vi "sv_Filter Even-Angle Signal for Specific Harmonic.vi"(0 "even-angle signals":cluster{"r0":dbl, "dr":dbl, "Y":dbl[]}[](array[cluster]), 2 "reset?":bool, 7 "even-angle position info":T1, 9 "specific harmonic":dbl=1.0 format="%0.2f", 11 "error in (no error)":errorcluster, 13 "zero delay? (F)":bool) -> (4 "even-angle signals out":cluster{"r0":dbl, "dr":dbl, "Y":dbl[]}[](array[cluster]), 8 "even-angle position info out":T1, 10 "phase delay [1/cycle]":dbl, 15 "error out":errorcluster)   [LabVIEW 2017, in "SoundVib_ContSweptSine.lvlib"]
uses:
  <vilib>/addons/Sound and Vibration/svt_Continuous Swept Sine/SoundVib_ContSweptSine.lvlib
  <vilib>/addons/Sound and Vibration/Order Analysis/Misc/OAT Position Info.ctl
  <vilib>/Analysis/3filter.llb/FIR Filter with I.C. (DBL).vi
  <vilib>/Analysis/NI_AALBase.lvlib
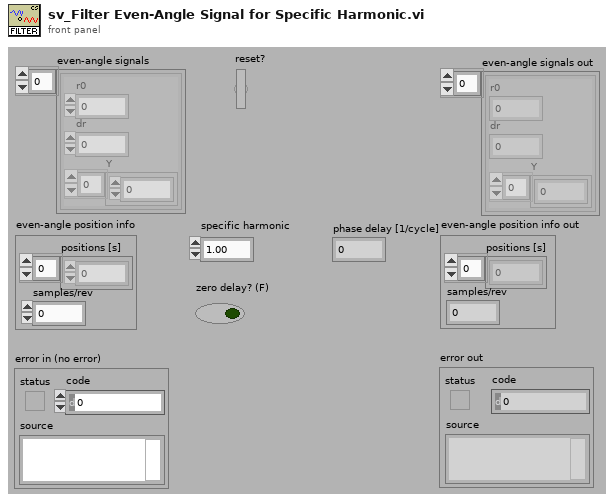
[diagram p1: front panel]
types:
  T1 = typedef "OAT Position Info.ctl" = cluster{"positions [s]":dbl[], "samples/rev":dbl}
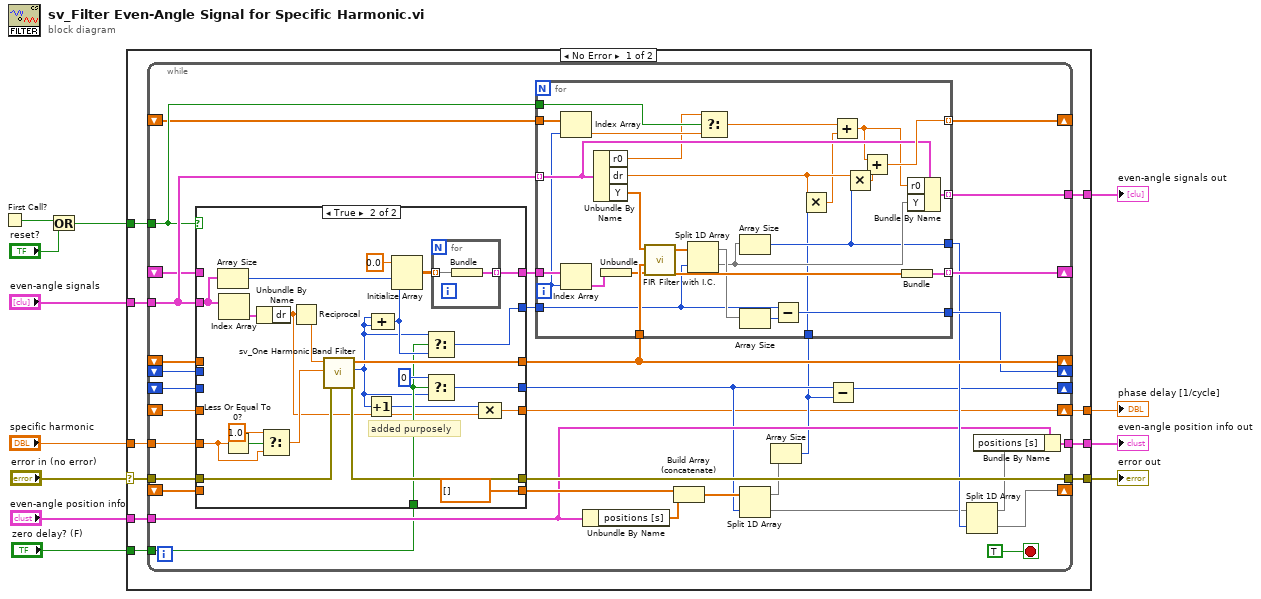
[diagram p0: block diagram]
diagram:
  n1 = First Call?() -> (First Call?: T/F=w12:bool)
  n2 = Or(x=w12, y="reset?") -> (x .or. y?=w10:bool)
  n3 = case shown="No Error" "error in (no error)" {
    selector: "error in (no error)" -> [w18 w121]
    tunnel: w10 -> [w22 _]
    tunnel: "even-angle signals" -> [w21 w120]
    tunnel: "specific harmonic" -> [w20 _]
    tunnel: [w19 w120] -> w7
    tunnel: [w17 w121] -> w5
    tunnel: "even-angle position info" -> [w16 w119]
    tunnel: [w15 w119] -> w3
    tunnel: "zero delay? (F)" -> [w14 _]
    tunnel: [w13 _] -> w1
    frame No Error {
      n4 = while {
        tunnel: w22 -> [w49]
        tunnel: w21 -> [w52]
        tunnel: w20 -> [w56]
        shift-right: [w51] -> _
        shift-left: _ -> [w55]
        shift-right: [w50] -> _
        shift-left: _ -> [w45]
        shift-right: [w53] -> _
        shift-left: _ -> [w44]
        shift-right: [w48] -> _
        shift-left: _ -> [w47]
        tunnel: [w46] -> w19
        tunnel: w18 -> [w43]
        tunnel: [w42] -> w17
        tunnel: w16 -> [w34]
        shift-right: [w39] -> _
        shift-left: _ -> [w38]
        tunnel: [w33] -> w15
        shift-right: [w29] -> _
        shift-left: _ -> [w28]
        tunnel: w14 -> [w27]
        shift-right: [w24] -> w13
        shift-left: _ -> [w23]
        stop <- TRUE stop-if-true
        n5 = case shown="True" w49 {
          tunnel: w52 -> [_ w112]
          tunnel: w56 -> [_ w105]
          tunnel: [w92 w114] -> w51
          tunnel: w55 -> [w92 _]
          tunnel: [w91 w109] -> w54
          tunnel: w45 -> [w87 _]
          tunnel: w44 -> [w91 _]
          tunnel: w43 -> [w90 w108]
          tunnel: [w90 w107] -> w42
          tunnel: w38 -> [w89 _]
          tunnel: [w89 dbl[] []] -> w36
          tunnel: [w88 w97] -> w32
          tunnel: w28 -> [w88 _]
          tunnel: w27 -> [_ w98]
          tunnel: [w87 w100] -> w26
          tunnel: [w86 w95] -> w24
          tunnel: w23 -> [w86 _]
          frame False {
          }
          frame True {
            # "added purposely"
            n6 = Array Size(array=w112) -> (size(s)=w111:i32)
            n7 = Index Array(array=w112) -> (element=w116:cluster{"r0":dbl, "dr":dbl, "Y":dbl[]})  [unwired: 1 in]
            n8 = Less Or Equal To 0?(x=w105) -> (x <= 0?=w106:bool)
            n9 = Unbundle By Name(w116) -> ("dr"=w96:dbl)
            n10 = Select(t=1.0, s=w106, f=w105) -> (s? t:f=w103:dbl)
            n11 = Reciprocal(x=w96) -> (1/x=w115:dbl)
            n12 = call <vilib>:"sv_One Harmonic Band Filter.vi"("error in (no error)"=w108, "specific harmonic"=w103, "fs"=w115) -> ("error out"=w107:errorcluster, "delay [samples]"=w94:i32, "FIR filter"=w114:dbl[])  [unwired: 6 in]
            n13 = Increment(x=w94) -> (x+1=w93:i32)
            n14 = Compound Arithmetic op=ADD(w94, w94) -> (w101:i32)
            n15 = Initialize Array(0.0 ("element"), w111, w101) -> (w110:dbl[][])
            n16 = Select(t=w94, s=w98, f=w101) -> (s? t:f=w100:i32)
            n17 = Select(t=0, s=w98, f=w94) -> (s? t:f=w97:i32)
            n18 = for {
              tunnel: w110 -> [w118] mode=indexing
              tunnel: [w117] -> w109 mode=indexing
              n19 = Bundle(w118) -> (w117:cluster{dbl[]})  [unwired: 1 in]
            }
            n20 = Compound Arithmetic op=MULTIPLY(w93, w96) -> (w95:dbl)
          }
        }
        n21 = Unbundle By Name(w34) -> ("positions [s]"=w41:dbl[])
        n22 = Build Array (concatenate)(w36, w41) -> (w37:dbl[])
        n23 = Split 1D Array(array=w37, index=w32) -> (first subarray=w30:dbl[], second subarray=w31:dbl[])
        n24 = Array Size(array=w30) -> (size(s)=w25:i32)
        n25 = for {
          tunnel: w54 -> [w85]
          tunnel: [w71] -> w53 mode=indexing
          tunnel: w52 -> [w76] mode=indexing
          tunnel: w51 -> [w82]
          tunnel: [w80] -> w50
          tunnel: w49 -> [w74]
          tunnel: [w77] -> w48 mode=indexing
          tunnel: w47 -> [w73]
          tunnel: [w72] -> w46 mode=indexing
          tunnel: [w66] -> w40
          tunnel: w26 -> [w65]
          tunnel: w25 -> [w63]
          i -> [w67]
          n26 = Index Array(array=w73, index=w67) -> (element=w69:dbl)
          n27 = Index Array(array=w85, index=w67) -> (element=w68:cluster{"Final X Conditions":dbl[]})
          n28 = Unbundle By Name(w76) -> ("r0"=w60:dbl, "dr"=w62:dbl, "Y"=w83:dbl[])
          n29 = Unbundle(w68) -> ("Final X Conditions"=w70:dbl[])
          n30 = call-poly <vilib>:"FIR Filter with I.C..vi"("Initial X Conditions"=w70, "FIR Coefficients"=w82, "X"=w83) -> ("Final X Conditions"=w84:dbl[], "Filtered X"=w81:dbl[])  [unwired: 5 in, 1 out]
          n31 = Split 1D Array(array=w81, index=w65) -> (first subarray=w79:dbl[], second subarray=w75:dbl[])
          n32 = Select(t=w60, s=w74, f=w69) -> (s? t:f=w59:dbl)
          n33 = Array Size(array=w75) -> (size(s)=w66:i32)
          n34 = Array Size(array=w79) -> (size(s)=w64:i32)
          n35 = Subtract(x=w65, y=w64) -> (x-y=w80:i32)
          n36 = Multiply(x=w62, y=w63) -> (x*y=w61:dbl)
          n37 = Add(x=w59, y=w61) -> (x+y=w58:dbl)
          n38 = Multiply(x=w62, y=w66) -> (x*y=w78:dbl)
          n39 = Add(x=w58, y=w78) -> (x+y=w77:dbl)
          n40 = Bundle("Final X Conditions"=w84) -> (w71:cluster{"Final X Conditions":dbl[]})  [unwired: 1 in]
          n41 = Bundle By Name(cluster=w76, "r0"=w58, "Y"=w75) -> (w72:cluster{"r0":dbl, "dr":dbl, "Y":dbl[]})
        }
        n42 = Subtract(x=w32, y=w25) -> (x-y=w29:i32)
        n43 = Split 1D Array(array=w31, index=w40) -> (first subarray=w35:dbl[], second subarray=w39:dbl[])
        n44 = Bundle By Name(cluster=w34, "positions [s]"=w35) -> (w33:T1)
      }
    }
    frame Error {
    }
  }
  "even-angle signals out" <- w7
  "error out" <- w5
  "even-angle position info out" <- w3
  "phase delay [1/cycle]" <- w1
